vi "B-Scan (Relative [FLR]) DVR.vi"(7 "Micropulse # In":i32, 9 "Scan definition":T1={"Scan Length"=0.0, "Inspection Resolution"=280.0, "Direction"=enum."Forwards"} {"Inspection Resolution" format="%#_6f"; "Scan Length" format="%#_6f"}, 10 "Axis No.":u8=1 min=1 max=4, 11 "scan data info":T3 {"Error Message" format="%04x"; "Message Header" format="%04x"; "IP"."MIP location" format="%#.0f"; "IP"."Location" format="%#.0f"; "PRF" format="%.0fHz"}) -> (0 "Update Display?":bool, 1 "B-Scan In Progress?":bool, 2 "B-Scan index":i32, 3 "data value reference":refnum<data-value>)   [LabVIEW 2026, in "MicroPulse_Driver.lvlib"]
uses:
  MicroPulse_Driver.lvlib
  Data/Datatypes/MP - scan data info.ctl
  Data/Datatypes/MP - data output format.ctl
  Data/Datatypes/MP - retain scan.ctl
  Data/Datatypes/MP - axis positions (LLC).ctl
  Data/Datatypes/MP - fly scan range (relative).ctl
  Data/Datatypes/MP - inspection direction (relative).ctl
  Low Level/FGV - B-Scan Active - Action [Enum].ctl
  <instrlib>/Micropulse/Micropulse.lvlib
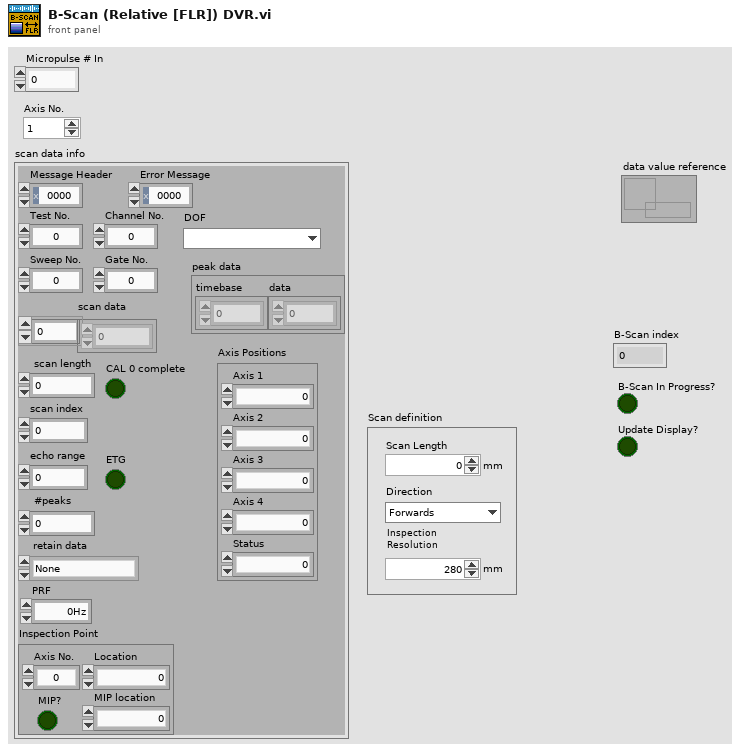
[diagram p1: front panel]
types:
  T1 = typedef "Micropulse.lvlib/MP - fly scan range (relative).ctl" = cluster{"Scan Length":dbl, "Inspection Resolution":dbl, "Direction":T2}
  T2 = typedef "Micropulse.lvlib/MP - inspection direction (relative).ctl" = enum16{"Forwards", "Backwards", "Bidirectional"}
  T3 = typedef "Micropulse.lvlib/MP - scan data info.ctl" = cluster{"Message Header":u16, "Error Message":u16, "Test No.":u32, "Channel No.":u8, "Sweep No.":u32, "Gate No.":u32, "DOF":T4, "retain data":T5, "scan data":u16[], "scan length":i32, "scan index":i32, "peak data":cluster{"timebase":u16[], "data":u16[]}, "#peaks":i32, "PRF":dbl, "IP":cluster{"Axis No.":u8, "Location":u32, "MIP location":u32, "MIP?":bool}, "echo range":u16, "ETG":bool, "CAL 0 complete":bool, "Axis Positions":T6}
  T4 = typedef "Micropulse.lvlib/MP - data output format.ctl" = enum16{"", "8-bit Mode", "10-bit Mode", "12-bit Mode", "16-bit Mode", "8-bit Log Mode", "12-bit Packed Mode"}
  T5 = typedef "Micropulse.lvlib/MP - retain scan.ctl" = enum16{"None", "Ascan", "Peaks"}
  T6 = typedef "Micropulse.lvlib/MP - axis positions (LLC).ctl" = cluster{"Axis 1":u32, "Axis 2":u32, "Axis 3":u32, "Axis 4":u32, "Status":u8}
  T7 = typedef "MicroPulse_Driver.lvlib/FGV - B-Scan Active - Action [Enum].ctl" = enum16{"Read", "Read & Reset Start Flag", "Start B-Scan", "B-Scan Finished"}
  T8 = cluster{"Lowest location":i32, "Highest location":i32}
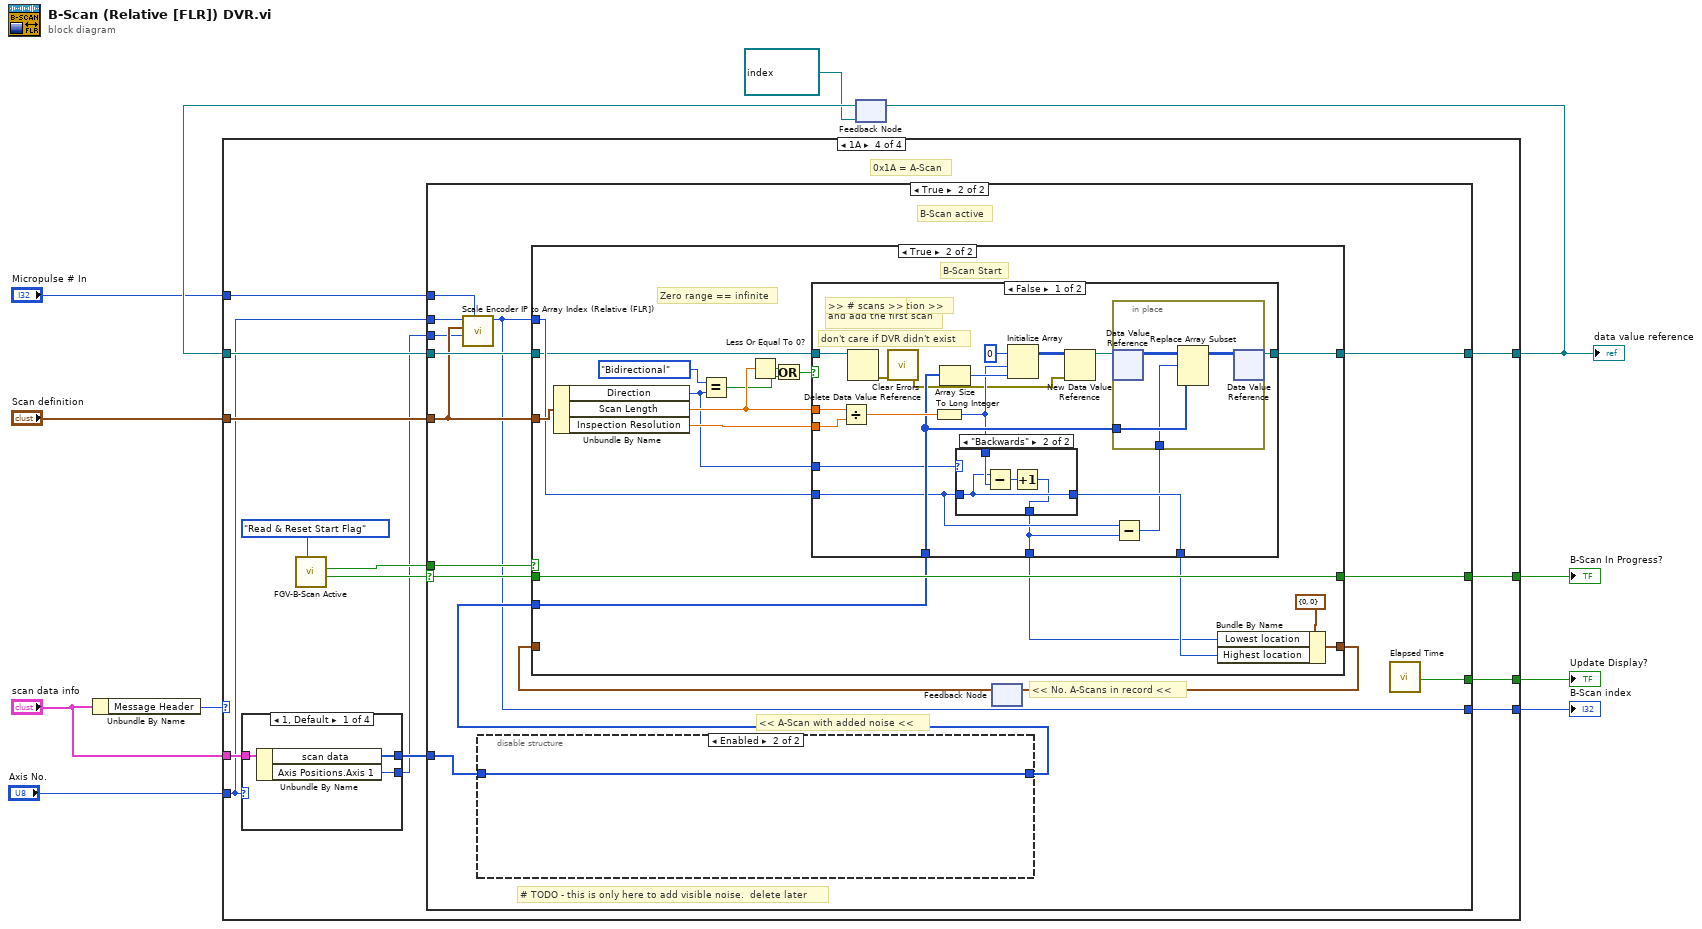
[diagram p0: block diagram]
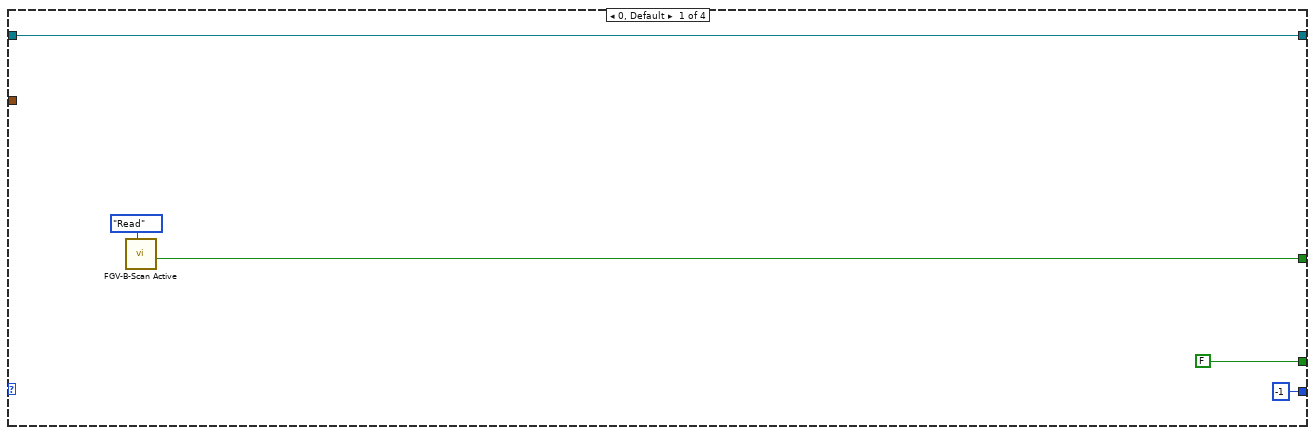
[diagram p2: hidden frame]
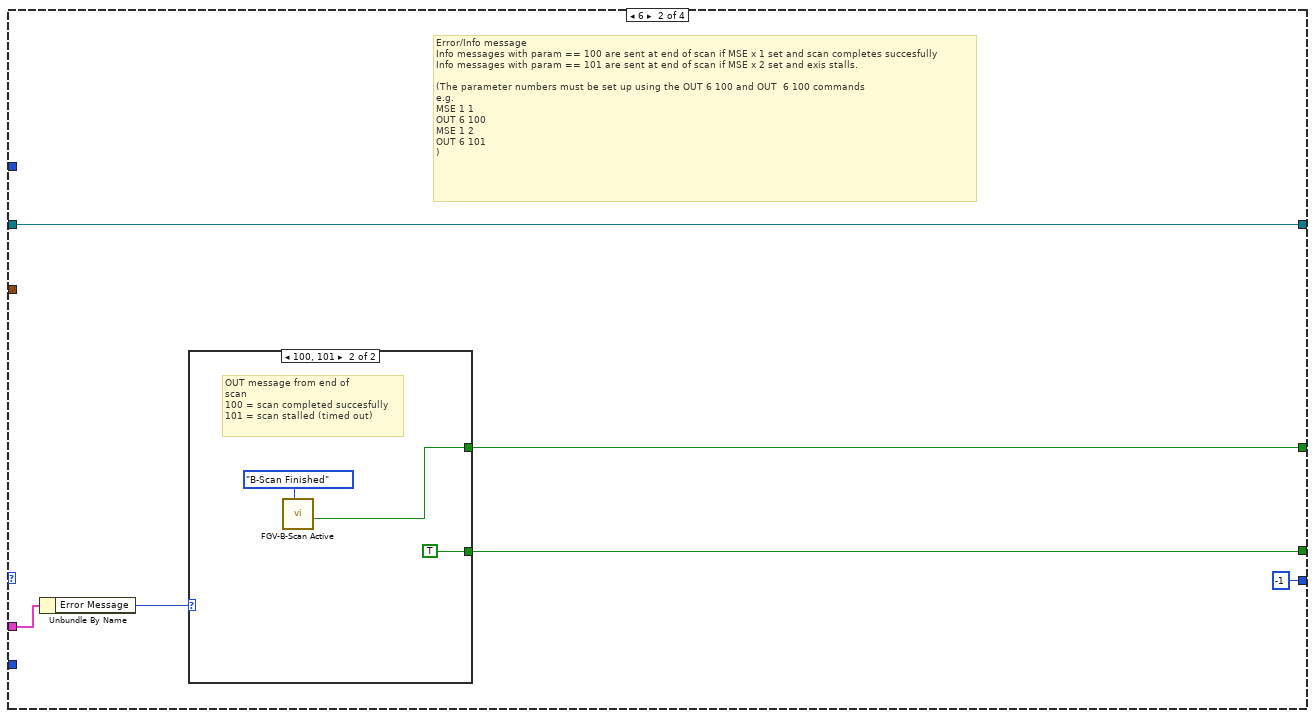
[diagram p3: hidden frame]
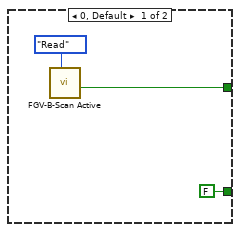
[diagram p4: hidden frame]
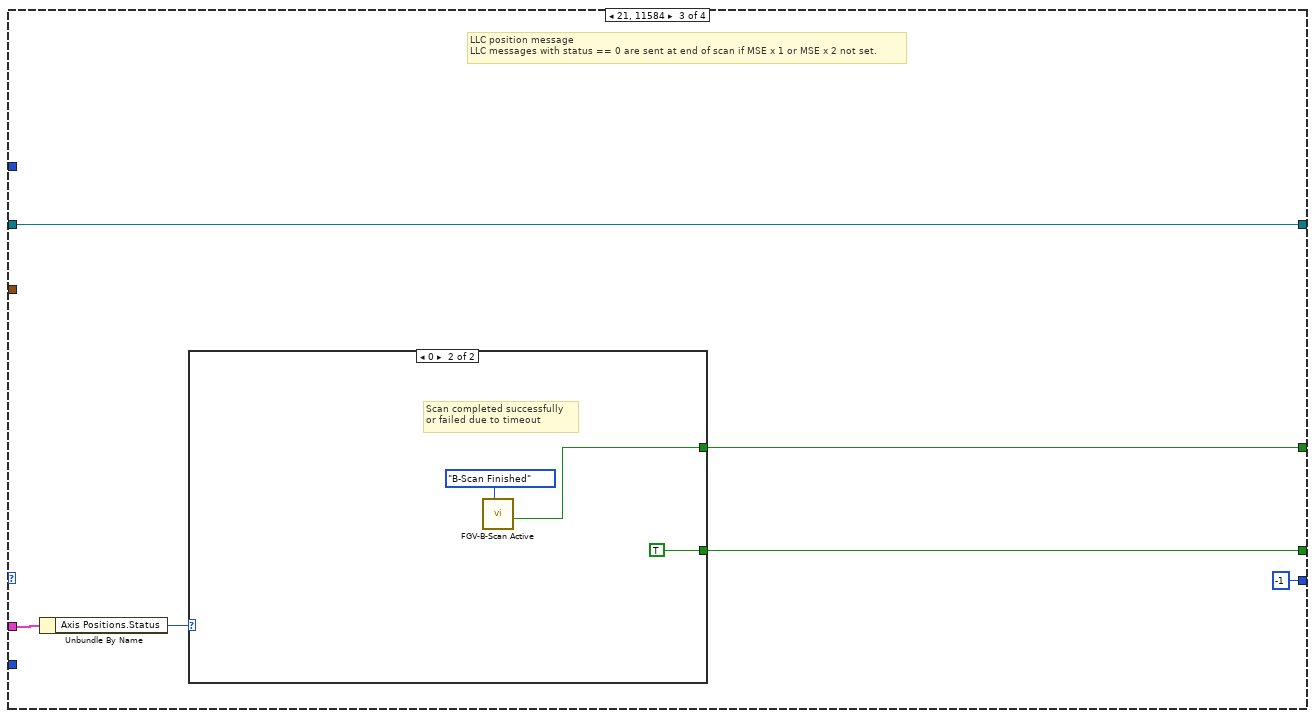
[diagram p5: hidden frame]
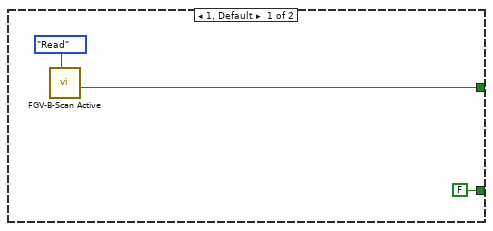
[diagram p6: hidden frame]
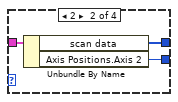
[diagram p7: hidden frame]
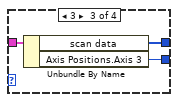
[diagram p8: hidden frame]
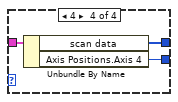
[diagram p9: hidden frame]
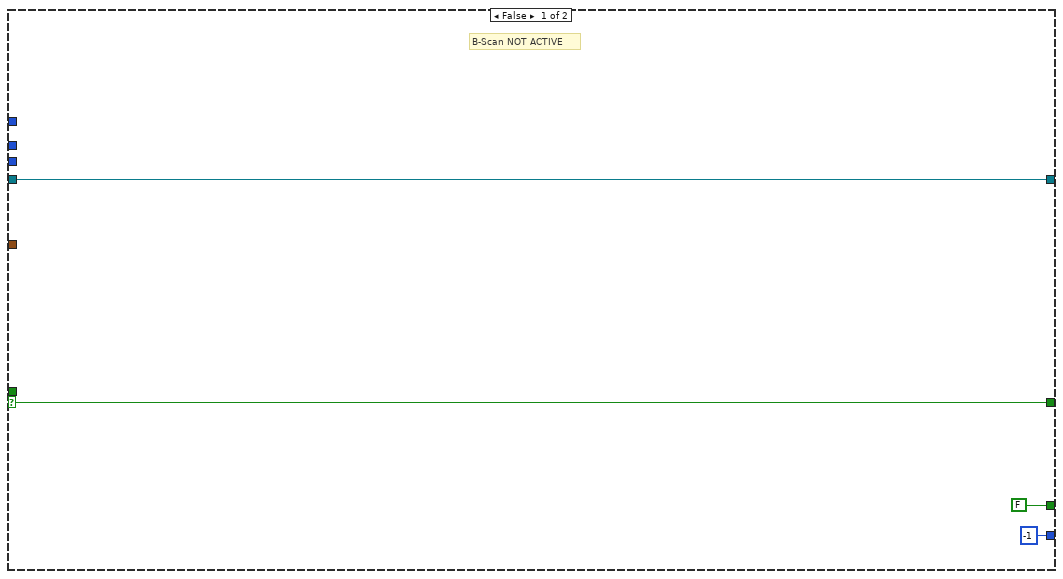
[diagram p10: hidden frame]
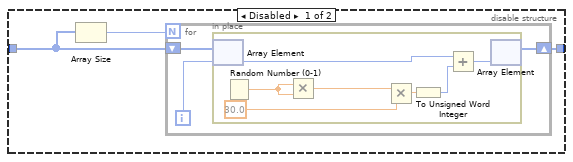
[diagram p11: hidden frame]
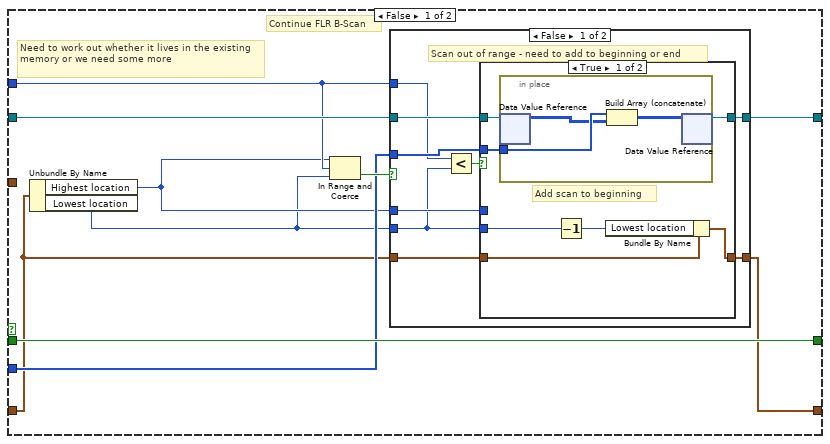
[diagram p12: hidden frame]
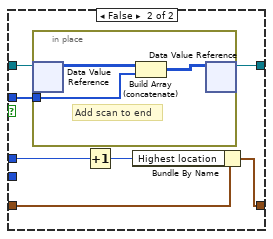
[diagram p13: hidden frame]
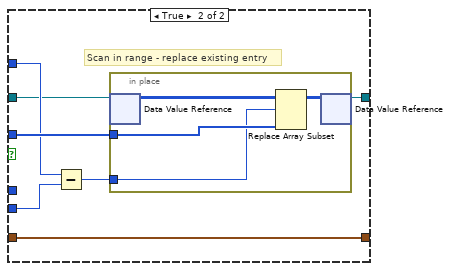
[diagram p14: hidden frame]
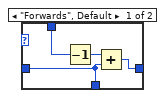
[diagram p15: hidden frame]
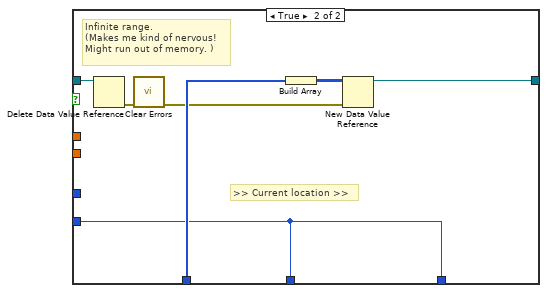
[diagram p16: hidden frame]
diagram:
  n1 = Unbundle By Name("scan data info") -> ("Message Header"=w11:u16)
  n2 = feedback #1(refnum<data-value> refnum ("data value reference")) -> (w7:refnum<data-value>)
  n3 = case shown="1A" w11 {
    tunnel: "scan data info" -> [_ w21 w33 w54]
    tunnel: "Scan definition" -> [_ _ _ w48]
    tunnel: [w16 w22 w34 w52] -> w8
    tunnel: w7 -> [w16 w22 w34 w51]
    tunnel: "Micropulse # In" -> [_ _ _ w47]
    tunnel: [w13 w19 w31 w50] -> w5
    tunnel: [FALSE w17 w29 w49] -> w4
    tunnel: "Axis No." -> [_ _ _ w42]
    tunnel: [-1 ("B-Scan index") -1 ("B-Scan index") -1 ("B-Scan index") w41] -> w2
    frame 0, Default {
      n4 = call "FGV-B-Scan Active.vi"("Action"=FGV_-_B-Scan_Active_-_Action_[Enum]."Read") -> ("B-Scan In Progress?"=w13:bool)  [unwired: 8 in, 2 out]
    }
    frame 6 {
      # "Error/Info message\nInfo messages with param == 100 are sent at end of scan if MSE x 1 set and scan completes succesfully\nInfo messages with param == 101 are sent at end of scan if MSE x 2 set and exis stalls.\n\n(The parameter numbers must be set up using the OUT 6 100 and OUT  6 100 commands \ne.g.\nMSE 1 1\nOUT 6 100\nMSE 1 2\nOUT 6 101\n)"
      n5 = Unbundle By Name(w21) -> ("Error Message"=w20:u16)
      n6 = case shown="100, 101" w20 {
        tunnel: [w24 w27] -> w19
        tunnel: [FALSE TRUE] -> w17
        frame 0, Default {
          n7 = call "FGV-B-Scan Active.vi"("Action"=FGV_-_B-Scan_Active_-_Action_[Enum]."Read") -> ("B-Scan In Progress?"=w24:bool)  [unwired: 8 in, 2 out]
        }
        frame 100, 101 {
          # "OUT message from end of\nscan\n100 = scan completed succesfully\n101 = scan stalled (timed out)"
          n8 = call "FGV-B-Scan Active.vi"("Action"=FGV_-_B-Scan_Active_-_Action_[Enum]."B-Scan Finished") -> ("B-Scan In Progress?"=w27:bool)  [unwired: 8 in, 2 out]
        }
      }
    }
    frame 21, 11584 {
      # "LLC position message\nLLC messages with status == 0 are sent at end of scan if MSE x 1 or MSE x 2 not set."
      n9 = Unbundle By Name(w33) -> ("Axis Positions.Status"=w32:u8)
      n10 = case shown="0" w32 {
        tunnel: [w36 w40] -> w31
        tunnel: [FALSE TRUE] -> w29
        frame 1, Default {
          n11 = call "FGV-B-Scan Active.vi"("Action"=FGV_-_B-Scan_Active_-_Action_[Enum]."Read") -> ("B-Scan In Progress?"=w36:bool)  [unwired: 8 in, 2 out]
        }
        frame 0 {
          # "Scan completed successfully\nor failed due to timeout"
          n12 = call "FGV-B-Scan Active.vi"("Action"=FGV_-_B-Scan_Active_-_Action_[Enum]."B-Scan Finished") -> ("B-Scan In Progress?"=w40:bool)  [unwired: 8 in, 2 out]
        }
      }
    }
    frame 26 {
      # "0x1A = A-Scan"
      n13 = case shown="1, Default" w42 {
        tunnel: w54 -> [w57 w60 w63 w66]
        tunnel: [w56 w59 w62 w65] -> w53
        tunnel: [w55 w58 w61 w64] -> w43
        frame 1, Default {
          n14 = Unbundle By Name(w57) -> ("scan data"=w56:u16[], "Axis Positions.Axis 1"=w55:u32)
        }
        frame 2 {
          n15 = Unbundle By Name(w60) -> ("scan data"=w59:u16[], "Axis Positions.Axis 2"=w58:u32)
        }
        frame 3 {
          n16 = Unbundle By Name(w63) -> ("scan data"=w62:u16[], "Axis Positions.Axis 3"=w61:u32)
        }
        frame 4 {
          n17 = Unbundle By Name(w66) -> ("scan data"=w65:u16[], "Axis Positions.Axis 4"=w64:u32)
        }
      }
      n18 = call "FGV-B-Scan Active.vi"("Action"=FGV_-_B-Scan_Active_-_Action_[Enum]."Read & Reset Start Flag") -> ("B-Scan In Progress?"=w44:bool, "B-Scan Start?"=w45:bool)  [unwired: 8 in, 1 out]
      n19 = case shown="True" w44 {
        selector: w44 -> [w69 w81]
        tunnel: w45 -> [_ w84]
        tunnel: w51 -> [w70 w85]
        tunnel: [w70 w79] -> w52
        tunnel: w53 -> [_ w78]
        tunnel: w48 -> [_ w75]
        tunnel: [w69 w82] -> w50
        tunnel: [FALSE w71] -> w49
        tunnel: w47 -> [_ w80]
        tunnel: w43 -> [_ w74]
        tunnel: w42 -> [_ w73]
        tunnel: [-1 ("B-Scan index") w72] -> w41
        frame False {
          # "B-Scan NOT ACTIVE"
        }
        frame True {
          # "<< A-Scan with added noise <<"
          # "B-Scan active"
          # "<< No. A-Scans in record <<"
          # "# TODO - this is only here to add visible noise.  delete later"
          n20 = call "Scale Encoder IP to Array Index (Relative (FLR]).vi"("Micropulse # In"=w80, "Inspection Point Location"=w74, "Scan definition"=w75, "Axis No."=w73) -> ("B-Scan index"=w72:i32)  [unwired: 7 in]
          n21 = disable-structure shown="Enabled" {
            disable-tunnel: w78 -> [w86 w99]
            disable-tunnel: [w87 w99] -> w77
            frame Disabled {
              n22 = Array Size(array=w86) -> (size(s)=w88:i32)
              n23 = for {
                N: w88 -> [_]
                shift-right: [w89] -> w87
                shift-left: w86 -> [w91]
                i -> [w90]
                n24 = in-place {
                  n25 = in-place-array #2(w91, w90) -> (w95:u16)
                  n26 = Random Number (0-1)() -> (number: 0 to 1=w92:dbl)
                  n27 = Multiply(x=w92, y=w92) -> (x*y=w93:dbl)
                  n28 = Multiply(x=w93, y=30.0) -> (x*y=w97:dbl)
                  n29 = To Unsigned Word Integer(number=w97) -> (unsigned 16bit integer=w96:u16)
                  n30 = Add(x=w95, y=w96) -> (x+y=w94:u16)
                  n31 = in-place-array #2(w94) -> (w89:u16[])  [unwired: 1 out]
                }
              }
            }
            frame Enabled {
            }
          }
          n32 = feedback #3() -> (w83:T8)  [unwired: 1 in]
          n33 = case shown="True" w84 {
            tunnel: w85 -> [w109 w151]
            tunnel: [w107 w150] -> w79
            tunnel: w75 -> [_ w166]
            tunnel: w72 -> [w105 w153]
            tunnel: w83 -> [w101 _]
            tunnel: [w108 w164] -> w82
            tunnel: w81 -> [w108 w164]
            tunnel: w77 -> [w104 w161]
            tunnel: [w100 w159] -> w76
            frame False {
              # "Continue FLR B-Scan"
              # "Need to work out whether it lives in the existing memory or we need some more"
              n34 = Unbundle By Name(w101) -> ("Highest location"=w103:i32, "Lowest location"=w102:i32)
              n35 = In Range and Coerce(upper limit=w103, x=w105, lower limit=w102) -> (In Range?=w106:bool)  [unwired: 1 out]
              n36 = case shown="False" w106 {
                tunnel: w109 -> [w118 w139]
                tunnel: [w117 w140] -> w107
                tunnel: w105 -> [w115 w144]
                tunnel: w104 -> [w116 w145]
                tunnel: w103 -> [w113 _]
                tunnel: w102 -> [w110 w141]
                tunnel: w101 -> [w112 w142]
                tunnel: [w111 w142] -> w100
                frame False {
                  # "Scan out of range - need to add to beginning or end"
                  n37 = Less?(x=w115, y=w110) -> (x < y?=w114:bool)
                  n38 = case shown="True" w114 {
                    tunnel: w118 -> [w120 w130]
                    tunnel: [w119 w129] -> w117
                    tunnel: w116 -> [w121 w135]
                    tunnel: w113 -> [_ w131]
                    tunnel: w110 -> [w124 _]
                    tunnel: w112 -> [w125 w134]
                    tunnel: [w122 w132] -> w111
                    frame True {
                      # "Add scan to beginning"
                      n39 = in-place {
                        in-place-border: w121 -> [w128]
                        n40 = in-place-dvr #4(w120) -> (w127:u16[][])  [unwired: 1 out]
                        n41 = Build Array (concatenate)(w128, w127) -> (w126:u16[][])
                        n42 = in-place-dvr #4(w126) -> (w119:refnum<data-value>)  [unwired: 1 out]
                      }
                      n43 = Decrement(x=w124) -> (x-1=w123:i32)
                      n44 = Bundle By Name(cluster=w125, "Lowest location"=w123) -> (w122:T8)
                    }
                    frame False {
                      n45 = in-place {
                        in-place-border: w135 -> [w138]
                        # "Add scan to end"
                        n46 = in-place-dvr #5(w130) -> (w136:u16[][])  [unwired: 1 out]
                        n47 = Build Array (concatenate)(w136, w138) -> (w137:u16[][])
                        n48 = in-place-dvr #5(w137) -> (w129:refnum<data-value>)  [unwired: 1 out]
                      }
                      n49 = Increment(x=w131) -> (x+1=w133:i32)
                      n50 = Bundle By Name(cluster=w134, "Highest location"=w133) -> (w132:T8)
                    }
                  }
                }
                frame True {
                  # "Scan in range - replace existing entry"
                  n51 = Subtract(x=w144, y=w141) -> (x-y=w143:i32)
                  n52 = in-place {
                    in-place-border: w145 -> [w149]
                    in-place-border: w143 -> [w148]
                    n53 = in-place-dvr #6(w139) -> (w146:u16[][])  [unwired: 1 out]
                    n54 = Replace Array Subset(array=w146, new element=w149, index (row)=w148) -> (w147:u16[][])  [unwired: 1 in]
                    n55 = in-place-dvr #6(w147) -> (w140:refnum<data-value>)  [unwired: 1 out]
                  }
                }
              }
            }
            frame True {
              # "Zero range == infinite"
              # "B-Scan Start"
              n56 = Unbundle By Name(w166) -> ("Direction"=w155:T2, "Scan Length"=w163:dbl, "Inspection Resolution"=w165:dbl)
              n57 = Equal?(x=MP_-_inspection_direction_(relative)."Bidirectional", y=w155) -> (x = y?=w156:bool)
              n58 = Less Or Equal To 0?(x=w163) -> (x <= 0?=w162:bool)
              n59 = Or(x=w162, y=w156) -> (x .or. y?=w157:bool)
              n60 = case shown="False" w157 {
                tunnel: [w167 w200] -> w150
                tunnel: w165 -> [w183 _]
                tunnel: w163 -> [w181 _]
                tunnel: w161 -> [w179 w203]
                tunnel: w153 -> [w176 w202]
                tunnel: w155 -> [w177 _]
                tunnel: [w175 w202] -> w154
                tunnel: [w174 w202] -> w152
                tunnel: w151 -> [w172 w199]
                frame False {
                  # "don't care if DVR didn't exist"
                  # ">> Current location >>"
                  # "Pre-allocate memory\nand add the first scan"
                  # ">> # scans >>"
                  n61 = Divide(x=w181, y=w183) -> (x/y=w182:dbl)
                  n62 = Delete Data Value Reference(data value reference=w172) -> (error out=w171:errorcluster)  [unwired: 1 in, 1 out]
                  n63 = call <vilib>:"Clear Errors.vi"("error in (no error)"=w171) -> ("error out"=w169:errorcluster)  [unwired: 5 in, 1 out]
                  n64 = To Long Integer(number=w182) -> (32bit integer=w178:i32)
                  n65 = Array Size(array=w179) -> (size(s)=w180:i32)
                  n66 = case shown="\"Backwards\"" w177 {
                    tunnel: w176 -> [w189 w194]
                    tunnel: w178 -> [w191 w196]
                    tunnel: [w190 w194] -> w175
                    tunnel: [w189 w193] -> w174
                    frame "Forwards", Default {
                      n67 = Decrement(x=w191) -> (x-1=w192:i32)
                      n68 = Add(x=w192, y=w189) -> (x+y=w190:i32)
                    }
                    frame "Backwards" {
                      n69 = Subtract(x=w194, y=w196) -> (x-y=w195:i32)
                      n70 = Increment(x=w195) -> (x+1=w193:i32)
                    }
                  }
                  n71 = Initialize Array(u16 0 ("index"), w178, w180) -> (w170:u16[][])
                  n72 = New Data Value Reference(data value=w170, error in=w169) -> (data value reference=w168:refnum<data-value>)  [unwired: 1 out]
                  n73 = Subtract(x=w176, y=w174) -> (x-y=w173:i32)
                  n74 = in-place {
                    in-place-border: w179 -> [w188]
                    in-place-border: w173 -> [w187]
                    n75 = in-place-dvr #7(w168) -> (w186:u16[][])  [unwired: 1 out]
                    n76 = Replace Array Subset(array=w186, new element=w188, index (row)=w187) -> (w185:u16[][])  [unwired: 1 in]
                    n77 = in-place-dvr #7(w185) -> (w167:refnum<data-value>)  [unwired: 1 out]
                  }
                }
                frame True {
                  # ">> Current location >>"
                  # "Infinite range.\n(Makes me kind of nervous!\nMight run out of memory. )"
                  n78 = Delete Data Value Reference(data value reference=w199) -> (error out=w198:errorcluster)  [unwired: 1 in, 1 out]
                  n79 = call <vilib>:"Clear Errors.vi"("error in (no error)"=w198) -> ("error out"=w197:errorcluster)  [unwired: 5 in, 1 out]
                  n80 = Build Array(w203) -> (w201:u16[][])
                  n81 = New Data Value Reference(data value=w201, error in=w197) -> (data value reference=w200:refnum<data-value>)  [unwired: 1 out]
                }
              }
              n82 = Bundle By Name(cluster=T8 {"Lowest location"=0, "Highest location"=0} ("input cluster"), "Lowest location"=w152, "Highest location"=w154) -> (w159:T8)
            }
          }
          n83 = feedback-in #3(w76) -> ()
          n84 = call "Elapsed Time"() -> ("Time has Elapsed"=w71:bool)  [unwired: 12 in, 7 out]
        }
      }
    }
  }
  "Update Display?" <- w4
  "B-Scan In Progress?" <- w5
  "B-Scan index" <- w2
  "data value reference" <- w8
  n85 = feedback-in #1(w8) -> ()
